vi "Get Signal Direction.vi"(8 "error in (no error)":errorcluster, 11 "Module in":refnum<class "Module.lvclass">) -> (0 "error out":errorcluster, 2 "Direction":enum16{"Input", "Output"}[](array[ring]), 3 "Module out":refnum<class "Module.lvclass">)   [LabVIEW 2015, in "Module.lvclass"]
uses:
  Module.lvclass
  IO/IO Class/Direction.ctl
  IO/IO Class/IO Class.lvclass
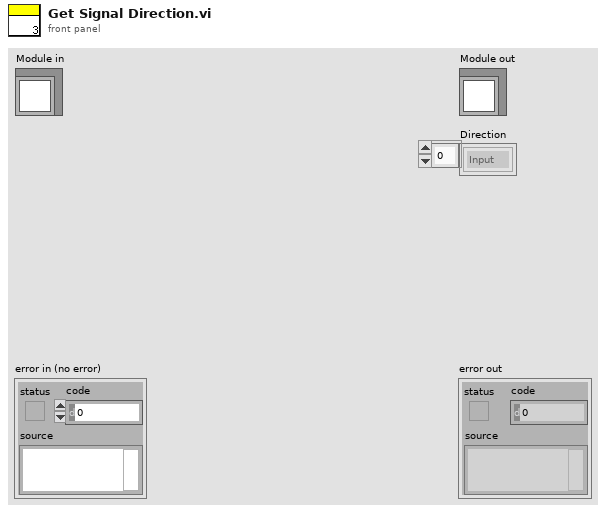
[diagram p1: front panel]
types:
  T1 = typedef "IO Class.lvclass/Direction.ctl" = cluster{"Direction":string}
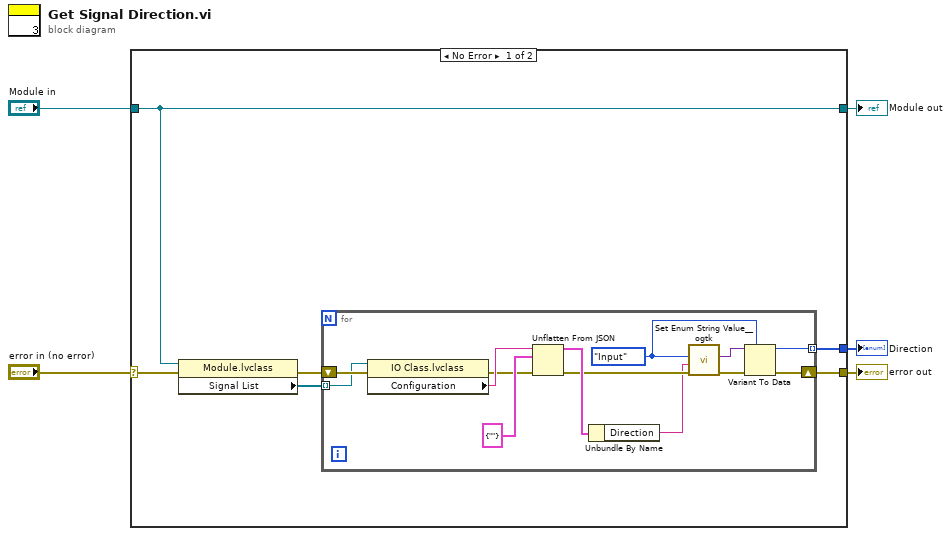
[diagram p0: block diagram]
diagram:
  n1 = case shown="No Error" "error in (no error)" {
    selector: "error in (no error)" -> [w10 w26]
    tunnel: [w7 w26] -> w4
    tunnel: [w11 w25] -> w2
    tunnel: "Module in" -> [w11 w25]
    tunnel: [w6 _] -> w1
    frame No Error {
      n2 = property class="Module.lvclass"(reference=w11, error in=w10) -> (error out=w9:errorcluster, "Signal List"=w8:refnum<class "IO Class.lvclass">[])  [unwired: 1 out]
      n3 = for {
        shift-right: [w15] -> w7
        shift-left: w9 -> [w24]
        tunnel: w8 -> [w23] mode=indexing
        tunnel: [w12] -> w6 mode=indexing
        w13 = enum16{"Input", "Output"}."Input" ("Direction")
        n4 = property class="IO Class.lvclass"(reference=w23, error in=w24) -> (error out=w20:errorcluster, "Configuration"=w22:string)  [unwired: 1 out]
        n5 = Unflatten From JSON(JSON string=w22, type and defaults=T1 {"Direction"=""} ("Cluster"), error in (no error)=w20) -> (value=w19:T1, error out=w18:errorcluster)  [unwired: 4 in]
        n6 = Unbundle By Name(w19) -> ("Direction"=w17:string)
        n7 = call <userlib>:"Set Enum String Value__ogtk.vi"("error in (no error)"=w18, "String Value"=w17, "Default Enum Value"=w13) -> ("error out"=w16:errorcluster, "Enum"=w14:variant)  [unwired: 7 in]
        n8 = Variant To Data(error in=w16, type=w13, Variant=w14) -> (data=w12:enum16{"Input", "Output"}, error out=w15:errorcluster)
      }
    }
    frame Error {
    }
  }
  "error out" <- w4
  "Module out" <- w2
  "Direction" <- w1
